vi "host.vi"() -> ()   [LabVIEW 2020]
uses:
  <vilib>/FPGAPlugInAG/cRIO-9035/niLvFpga_Open_cRIO-9035.vi
  <vilib>/rvi/interface/common/dynamic/niFpgaDynamicAddResources.vi
  <vilib>/Utility/error.llb/Error Cluster From Error Code.vi
  <vilib>/rvi/errors/niLvFpgaAdjustHostInterfaceError.vi
  <vilib>/FPGAPlugInAG/Dynamic/niLvFpga_Run_Dynamic.vi
  <vilib>/FPGAPlugInAG/Dynamic/niLvFpga_Close_Dynamic.vi
  <vilib>/rvi/interface/nirviOpenFPGA/nirviOpenFPGA.xnode
  FPGA Bitfiles/fftfpgaapplicati_FPGATarget_FFT2_9G-jDMvWUhs.lvbitx
  FFT.vi
  <vilib>/rvi/interface/nirviMethod/nirviMethod.xnode
  <vilib>/rvi/interface/nirviCloseFPGA/nirviCloseFPGA.xnode
  <vilib>/rvi/errors/niLvFpgaMergeErrorWithErrorCode.vi
  <vilib>/FPGAPlugInAG/Dynamic/niLvFpga_ReadFifo_Dynamic.vi
  <vilib>/Analysis/NI_AALPro.lvlib
  <vilib>/FPGAPlugInAG/Dynamic/niLvFpga_WriteFifo_Dynamic.vi
panel:
  out "start tick I32":i32[](array[numeric])
  out "end tick I32":i32[](array[numeric])
  out "index case":i32
  out "index":i32
  out "indexcase":fxp<+/-,32,16>[](array[numeric])
  out "index":fxp<+/-,32,16>[](array[numeric])
  out "real array size":i32
  out "imaginaryDBL array size":i32
  out "real Fixed":fxp<+/-,32,21>[](array[numeric])
  out "imaginary Fixed":fxp<+/-,32,21>[](array[numeric])
  out "imaginary number DBL from FIFO":dbl[](array[numeric])
  out "real number DBL  from FIFO":dbl[](array[numeric])
  out "detrend acc":dbl[](graph)
  out "acc":dbl[](graph)
  out "samples":i32
  out "Array":fxp<+/-,32,16>[](array[numeric])
  out "end tick":fxp<+/-,32,16>[](array[numeric])
  out "start ticka":fxp<+/-,32,16>[](array[numeric])
  out "Waveform Graph":dbl[][](graph)
  out "input signal":T1(graph)
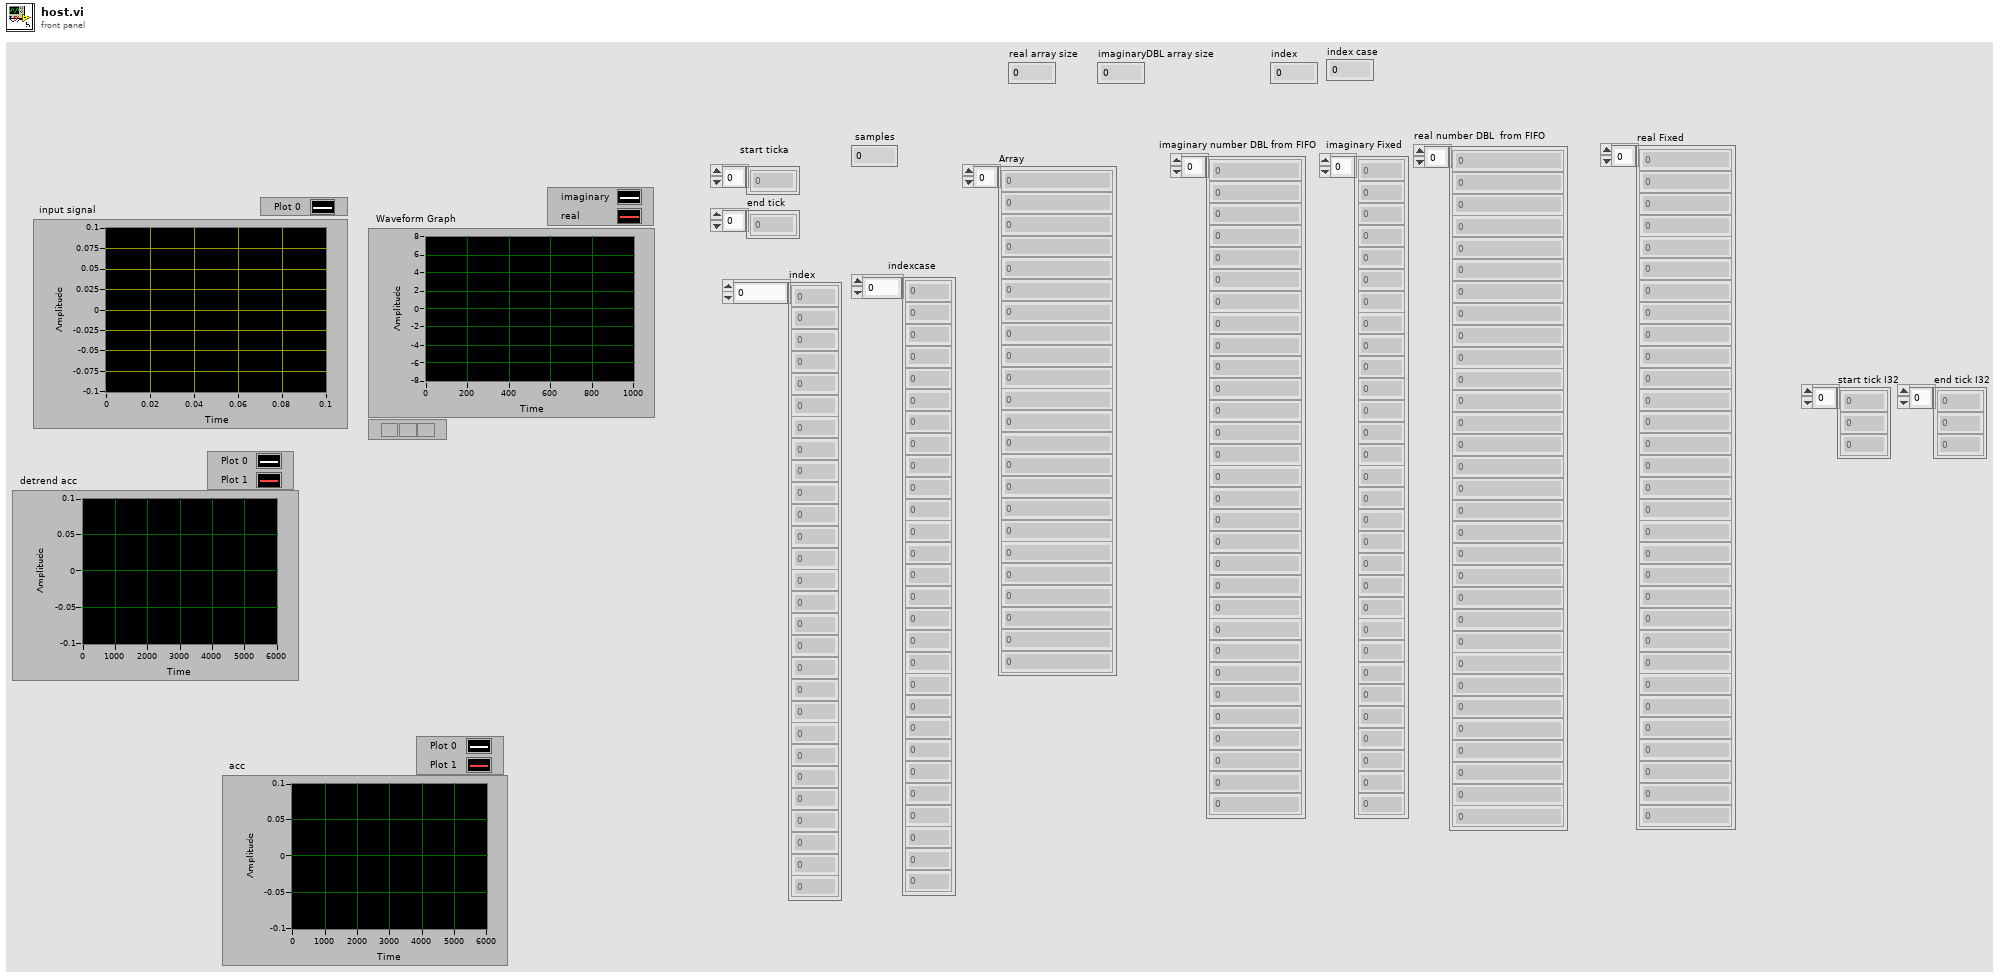
[diagram p1: front panel]
types:
  T1 = cluster{"array type (2D Dbl)":dbl[], "array type (2D Dbl)":dbl[]}
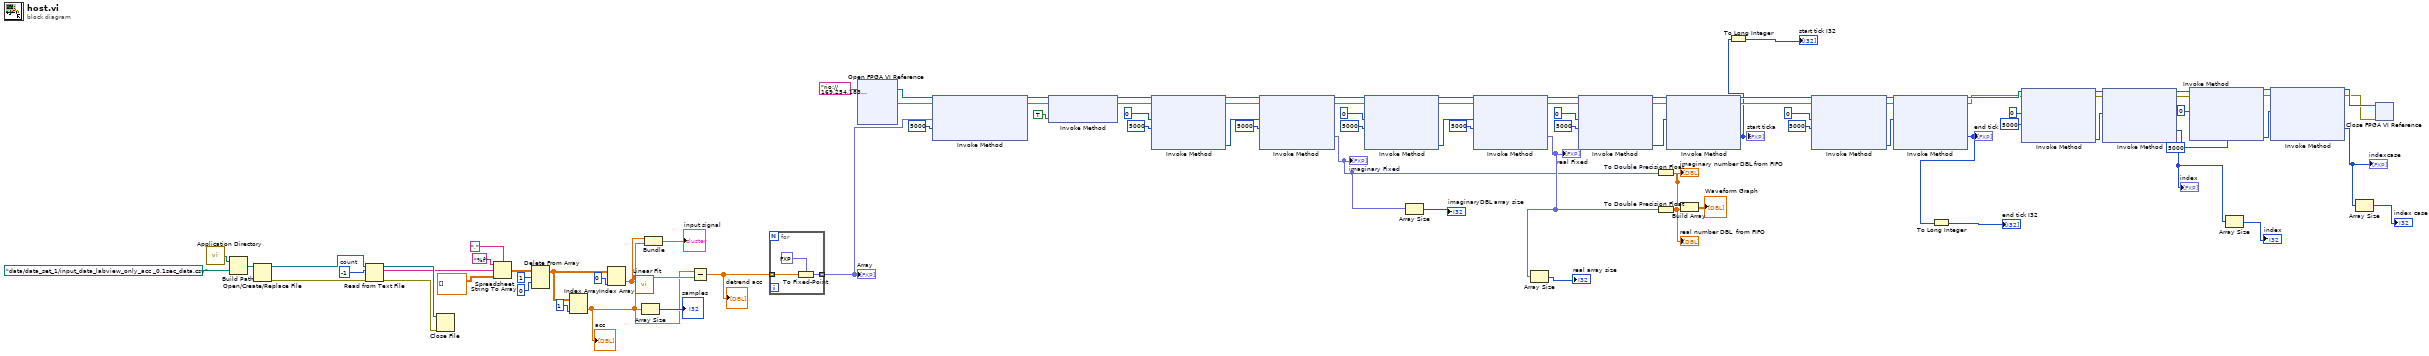
[diagram p0: block diagram]
diagram:
  w84 = -1  # count
  n1 = call <vilib>:"Application Directory.vi"() -> ("Application Directory"=w88:path)
  n2 = Build Path(base path=w88, name or relative path=path "data/data_set_1/input_data_labview_only_acc _0.1sec_data.csv" ("default name")) -> (appended path=w87:path)
  n3 = Open/Create/Replace File(file path (use dialog)=w87) -> (refnum out=w92:refnum<file>, error out=w93:errorcluster)  [unwired: 5 in, 1 out]
  n4 = Read from Text File(file (use dialog)=w92, count=w84, error in=w93) -> (refnum out=w91:refnum<file>, text=w89:string, error out=w90:errorcluster)  [unwired: 1 in, 1 out]
  n5 = Close File(refnum=w91, error in=w90) -> ()  [unwired: 2 out]
  n6 = Spreadsheet String To Array(delimiter (Tab)=",", format string="%f", spreadsheet string=w89, array type (2D Dbl)=dbl[][] []) -> (array=w81:dbl[][])
  n7 = Delete From Array(array=w81, length=1, index (row)=0) -> (array with subset deleted=w76:dbl[][])  [unwired: 1 in, 1 out]
  n8 = Index Array(array=w76, index (col)=1 ("disabled index (col)")) -> (element=w31:dbl[])  [unwired: 1 in]
  "acc" <- w31
  n9 = Index Array(array=w76, index (col)=0 ("disabled index (col)")) -> (element=w34:dbl[])  [unwired: 1 in]
  n10 = call <vilib>:"Linear Fit.vi"("Y"=w31, "X"=w34) -> ("Best Linear Fit"=w32:dbl[])  [unwired: 9 in, 4 out]
  n11 = Array Size(array=w31) -> (size(s)=→"samples":i32)
  n12 = Bundle("array type (2D Dbl)"=w34, "array type (2D Dbl)"=w31) -> (→"input signal":T1)  [unwired: 1 in]
  n13 = Subtract(x=w31, y=w32) -> (x-y=w33:dbl[])
  "detrend acc" <- w33
  n14 = for {
    tunnel: [w95] -> w36 mode=indexing
    tunnel: w33 -> [w94] mode=indexing
    n15 = To Fixed-Point(fixed-point type=fxp<+/-,32,16> 0.0 ("f"), number=w94) -> (fixed-point=w95:fxp<+/-,32,16>)
  }
  "Array" <- w36
  n16 = xnode "Open FPGA VI Reference"("resource name"=tag "rio://169.254.183.73/RIO0") -> ("FPGA VI Reference Out"=w74:refnum<k20>, "error out"=w73:errorcluster)  [unwired: 1 in]
  n17 = xnode "Invoke Method"("FPGA VI Reference In"=w74, "error in"=w73, "Data"=w36, "Timeout (ms)"=5000) -> ("FPGA VI Reference Out"=w71:refnum<k20>, "error out"=w70:errorcluster)  [unwired: 1 out]
  n18 = xnode "Invoke Method"("FPGA VI Reference In"=w71, "error in"=w70, "Wait Until Done (F)"=TRUE) -> ("FPGA VI Reference Out"=w69:refnum<k20>, "error out"=w68:errorcluster)
  n19 = xnode "Invoke Method"("FPGA VI Reference In"=w69, "error in"=w68, "Number of Elements"=u32 0, "Timeout (ms)"=5000) -> ("FPGA VI Reference Out"=w67:refnum<k20>, "error out"=w66:errorcluster, "Elements Remaining"=w60:u32)  [unwired: 1 out]
  n20 = xnode "Invoke Method"("FPGA VI Reference In"=w67, "error in"=w66, "Number of Elements"=w60, "Timeout (ms)"=5000) -> ("FPGA VI Reference Out"=w63:refnum<k20>, "error out"=w62:errorcluster, "Data"=w3:fxp<+/-,32,16>[])  [unwired: 1 out]
  "imaginary Fixed" <- w3
  n21 = xnode "Invoke Method"("FPGA VI Reference In"=w63, "error in"=w62, "Number of Elements"=u32 0, "Timeout (ms)"=5000) -> ("FPGA VI Reference Out"=w65:refnum<k20>, "error out"=w64:errorcluster, "Elements Remaining"=w58:u32)  [unwired: 1 out]
  n22 = Array Size(array=w3) -> (size(s)=→"imaginaryDBL array size":i32)
  n23 = xnode "Invoke Method"("FPGA VI Reference In"=w65, "error in"=w64, "Number of Elements"=w58, "Timeout (ms)"=5000) -> ("FPGA VI Reference Out"=w55:refnum<k20>, "error out"=w54:errorcluster, "Data"=w4:fxp<+/-,32,16>[])  [unwired: 1 out]
  "real Fixed" <- w4
  n24 = Array Size(array=w4) -> (size(s)=→"real array size":i32)
  n25 = xnode "Invoke Method"("FPGA VI Reference In"=w55, "error in"=w54, "Number of Elements"=u32 0, "Timeout (ms)"=5000) -> ("FPGA VI Reference Out"=w53:refnum<k20>, "error out"=w52:errorcluster, "Elements Remaining"=w47:u32)  [unwired: 1 out]
  n26 = To Double Precision Float(number=w3) -> (double precision float=w1:dbl[])
  "imaginary number DBL from FIFO" <- w1
  n27 = To Double Precision Float(number=w4) -> (double precision float=w2:dbl[])
  "real number DBL  from FIFO" <- w2
  n28 = xnode "Invoke Method"("FPGA VI Reference In"=w53, "error in"=w52, "Number of Elements"=w47) -> ("FPGA VI Reference Out"=w51:refnum<k20>, "error out"=w50:errorcluster, "Data"=w5:u32[])  [unwired: 1 in, 1 out]
  "start ticka" <- w5
  n29 = Build Array(w1, w2) -> (→"Waveform Graph":dbl[][])
  n30 = To Long Integer(number=w5) -> (32bit integer=→"start tick I32":i32[])
  n31 = xnode "Invoke Method"("FPGA VI Reference In"=w51, "error in"=w50, "Number of Elements"=u32 0, "Timeout (ms)"=5000) -> ("FPGA VI Reference Out"=w49:refnum<k20>, "error out"=w48:errorcluster, "Elements Remaining"=w45:u32)  [unwired: 1 out]
  n32 = xnode "Invoke Method"("FPGA VI Reference In"=w49, "error in"=w48, "Number of Elements"=w45) -> ("FPGA VI Reference Out"=w28:refnum<k20>, "error out"=w27:errorcluster, "Data"=w9:u32[])  [unwired: 1 in, 1 out]
  "end tick" <- w9
  n33 = To Long Integer(number=w9) -> (32bit integer=→"end tick I32":i32[])
  n34 = xnode "Invoke Method"("FPGA VI Reference In"=w28, "error in"=w27, "Number of Elements"=u32 0, "Timeout (ms)"=5000) -> ("FPGA VI Reference Out"=w26:refnum<k20>, "error out"=w25:errorcluster, "Elements Remaining"=w16:u32)  [unwired: 1 out]
  n35 = xnode "Invoke Method"("FPGA VI Reference In"=w26, "error in"=w25, "Number of Elements"=w16) -> ("FPGA VI Reference Out"=w24:refnum<k20>, "error out"=w23:errorcluster, "Data"=w8:u16[])  [unwired: 1 in, 1 out]
  "index" <- w8
  n36 = xnode "Invoke Method"("FPGA VI Reference In"=w24, "error in"=w23, "Number of Elements"=u32 0, "Timeout (ms)"=5000) -> ("FPGA VI Reference Out"=w22:refnum<k20>, "error out"=w20:errorcluster, "Elements Remaining"=w13:u32)  [unwired: 1 out]
  n37 = Array Size(array=w8) -> (size(s)=→"index":i32)
  n38 = xnode "Invoke Method"("FPGA VI Reference In"=w22, "error in"=w20, "Number of Elements"=w13) -> ("FPGA VI Reference Out"=w21:refnum<k20>, "error out"=w19:errorcluster, "Data"=w7:u16[])  [unwired: 1 in, 1 out]
  "indexcase" <- w7
  n39 = Array Size(array=w7) -> (size(s)=→"index case":i32)
  n40 = xnode "Close FPGA VI Reference"("FPGA VI Reference In"=w21, "error in"=w19) -> ()  [unwired: 1 out]
